vi "Dark Theme Message Style.vi"() -> (0 "Text Style":T1={"Text Formatting"={"Font"="", "Text Color"=enum."Black", "Background Color"=enum."White", "Style"=enum."Regular", "Font Size"=10.0, "Alignment"=enum."Left"}, "Text Style Name"="Message"} {"Text Formatting"."Font Size" min=6.0 step=1.0})   [LabVIEW 2021, in "Notebook.lvlib"]
uses:
  Named Text Style.ctl
  Text Formatting.ctl
  Text Colors.ctl
  Text Style.ctl
  Text Alignment.ctl
  Notebook/Notebook.lvlib
  Rich Text Box.lvlib
panel:
  # "see the License on the block diagram (Ctrl+E or Window:Show Block Diagram)"
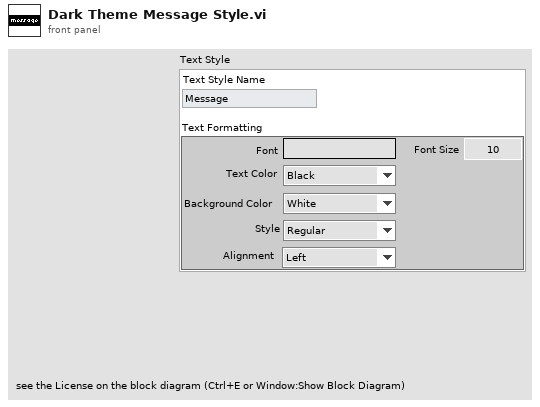
[diagram p1: front panel]
types:
  T1 = typedef "Notebook.lvlib/Named Text Style.ctl" = cluster{"Text Formatting":T2, "Text Style Name":string}
  T2 = typedef "Rich Text Box.lvlib/Text Formatting.ctl" = cluster{"Font":string, "Text Color":T3, "Background Color":T3, "Style":T4, "Font Size":dbl, "Alignment":T5}
  T3 = typedef "Rich Text Box.lvlib/Text Colors.ctl" = enum16{"Unchanged", "Black", "Blue", "Cyan", "Maroon", "Gray", "Violet", "Green", "Light Green", "Orange", "Yellow", "Magenta", "Red", "White"}
  T4 = typedef "Rich Text Box.lvlib/Text Style.ctl" = enum16{"Regular", "Bold", "Italic", "Underline", "Strikeout"}
  T5 = typedef "Rich Text Box.lvlib/Text Alignment.ctl" = enum16{"Left", "Right", "Center"}
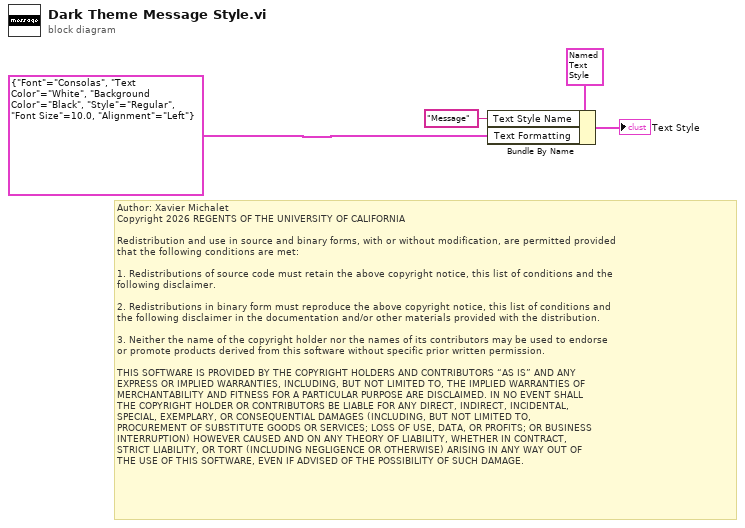
[diagram p0: block diagram]
diagram:
  # "Author: Xavier Michalet\nCopyright 2026 REGENTS OF THE UNIVERSITY OF CALIFORNIA\n\nRedistribution and use in source and binary forms, with or without modification, are permitted provided\nthat the following conditions are met:\n\n1. Redistributions of source code must retain the above copyright notice, this list of conditions and the\nfollowing disclaimer.\n\n2. Redistributions in binary form must reproduce the above copyright notice, this list of conditions and\nthe following disclaimer in the documentation and/or other materials provided with the distribution.\n\n3. Neither the name of the copyright holder nor the names of its contributors may be used to endorse \nor promote products derived from this software without specific prior written permission.\n\nTHIS SOFTWARE IS PROVIDED BY THE COPYRIGHT HOLDERS AND CONTRIBUTORS “AS IS” AND ANY \nEXPRESS OR IMPLIED WARRANTIES, INCLUDING, BUT NOT LIMITED TO, THE IMPLIED WARRANTIES OF\nMERCHANTABILITY AND FITNESS FOR A PARTICULAR PURPOSE ARE DISCLAIMED. IN NO EVENT SHALL\nTHE COPYRIGHT HOLDER OR CONTRIBUTORS BE LIABLE FOR ANY DIRECT, INDIRECT, INCIDENTAL, \nSPECIAL, EXEMPLARY, OR CONSEQUENTIAL DAMAGES (INCLUDING, BUT NOT LIMITED TO, \nPROCUREMENT OF SUBSTITUTE GOODS OR SERVICES; LOSS OF USE, DATA, OR PROFITS; OR BUSINESS\nINTERRUPTION) HOWEVER CAUSED AND ON ANY THEORY OF LIABILITY, WHETHER IN CONTRACT, \nSTRICT LIABILITY, OR TORT (INCLUDING NEGLIGENCE OR OTHERWISE) ARISING IN ANY WAY OUT OF\nTHE USE OF THIS SOFTWARE, EVEN IF ADVISED OF THE POSSIBILITY OF SUCH DAMAGE."
  n1 = Bundle By Name(cluster=T1 {"Text Formatting"={"Font"="", "Text Color"=enum."Black", "Background Color"=enum."White", "Style"=enum."Regular", "Font Size"=10.0, "Alignment"=enum."Left"}, "Text Style Name"="Message"} ("Text Style"), "Text Style Name"="Message", "Text Formatting"=T2 {"Font"="Consolas", "Text Color"=enum."White", "Background Color"=enum."Black", "Style"=enum."Regular", "Font Size"=10.0, "Alignment"=enum."Left"} ("Default Text Formatting")) -> (→"Text Style":T1)
